vi "Set UI VI Reference.vi"(8 "error in (no error)":errorcluster, 10 "UI VI Reference (caller)":refnum<vi>, 11 "Flex UI (Actor) in":refnum<class "Flex UI (Actor).lvclass">) -> (0 "error out":errorcluster, 3 "Flex UI (Actor) out":refnum<class "Flex UI (Actor).lvclass">)   [LabVIEW 2016, in "Flex UI (Parent Actor).lvlib" / "Flex UI (Actor).lvclass"]
doc: "Wrapper around the Set UI VI Reference method within the Flex UI class. This sets the UI VI Reference that resides in the private data of the Flex UI class."
uses:
  Flex UI (Actor).lvclass
  <vilib>/East West Architects/Flex UI/Flex UI (Parent)/Flex UI.lvclass
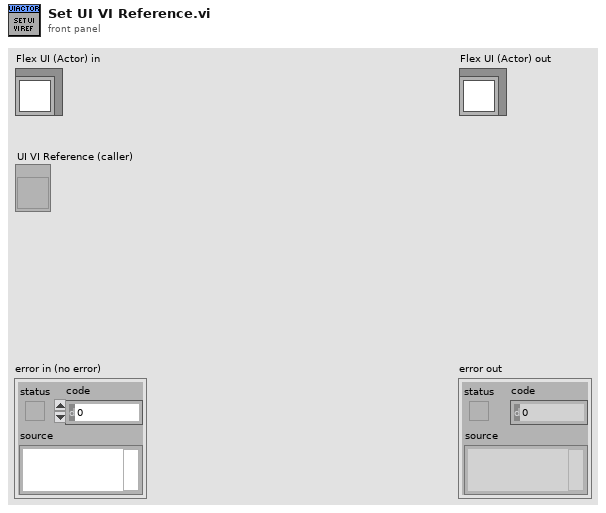
[diagram p1: front panel]
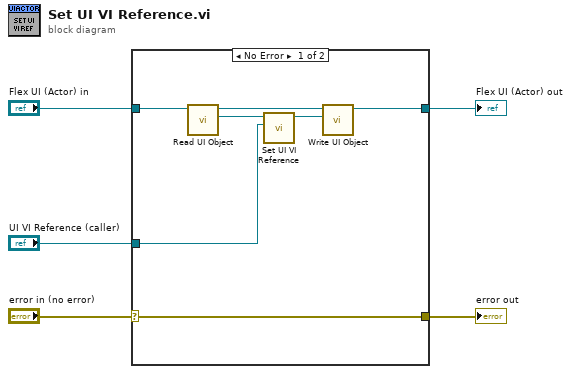
[diagram p0: block diagram]
diagram:
  n1 = case shown="No Error" "error in (no error)" {
    selector: "error in (no error)" -> [w11 w14]
    tunnel: [w11 w14] -> w4
    tunnel: [w9 w13] -> w2
    tunnel: "Flex UI (Actor) in" -> [w12 w13]
    tunnel: "UI VI Reference (caller)" -> [w6 _]
    frame No Error {
      n2 = call-dynamic "Read UI Object.vi"("Flex UI (Actor) in"=w12) -> ("Flex UI Object"=w8:refnum<class "Flex UI.lvclass">, "Flex UI (Actor) out"=w10:refnum<class "Flex UI (Actor).lvclass">)  [unwired: 8 in, 1 out]
      n3 = call-dynamic "Set UI VI Reference.vi"("UI VI Reference (caller)"=w6, "Flex UI in"=w8) -> ("Flex UI out"=w7:refnum<class "Flex UI.lvclass">)  [unwired: 8 in, 1 out]
      n4 = call-dynamic "Write UI Object.vi"("Flex UI in"=w7, "Flex UI (Actor) in"=w10) -> ("Flex UI (Actor) out"=w9:refnum<class "Flex UI (Actor).lvclass">)  [unwired: 8 in, 1 out]
    }
    frame Error {
    }
  }
  "error out" <- w4
  "Flex UI (Actor) out" <- w2
